vi "Graph Events.vi"() -> ()   [LabVIEW 2023]
doc: "This example shows some of the Waveform Graph events including cursor movement and changes in graph scale and plot properties."
panel:
  out "Iteration":i32
  out "Event Captured":string
  in  "Stop":bool
  out "Graph":dbl[](graph)
  # "Overview: Demonstrates several Events specific to graph indicators.\nInstructions:\n1. Run the VI and observe the Event Captured value when performing the following steps.\n2. Move the cursor within the graph.\n3. Click the image in the plot legend and select Common Plots, then select a new plot style.\n4. Change the minimum and/or maximum values in the X and Y scales.\n5. Click Stop to stop the VI."
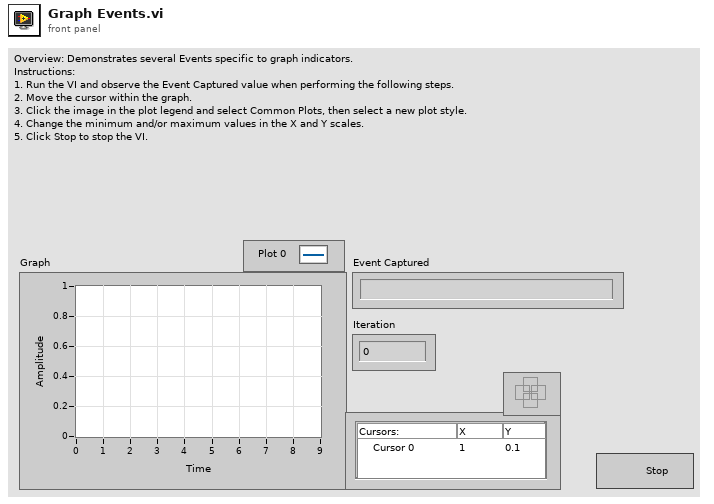
[diagram p1: front panel]
types:
  T1 = typedef "lveventtype.ctl" = enum32{"Null", "Timeout", "Annotation Menu Selection", "Annotation Menu Selection?", "App Instance Close", "App Instance Close?", "Autoscale Range Change", "Bookmark Info Change", "Cell Edit", "Cell Edit?", "Cursor Grab", "Cursor Grab?", "Cursor Menu Selection", "Cursor Menu Selection?", "Cursor Move", "Cursor Release", "Data Change", "Direction Change", "Display State Change", "Drag Ended", "Drag Enter", "Drag Leave", "Drag Over", "Drag Source Update", "Drag Starting", "Drag Starting?", "Drop", "Exec State Change", "Key Down", "Key Down?", "Key Repeat", "Key Repeat?", "Key Up", "Listbox Double Click", "Menu Activation?", "Menu Selection (App)", "Menu Selection? (App)", "Menu Selection (User)", "Mouse Down", "Mouse Down?", "Mouse Enter", "Mouse Leave", "Mouse Move", "Mouse Up", "Mouse Wheel", "NI Security User Change (App)", "Pane Size", "Panel Close", "Panel Close?", "Panel Resize", "Plot Attribute Change", "Scale Range Change", "Shortcut Menu Activation?", "Shortcut Menu Selection (App)", "Shortcut Menu Selection? (App)", "Shortcut Menu Selection (User)", "Tree Double Click", "Tree Drag", "Tree Drag?", "Tree Drop", "Tree Drop?", "Tree Item Close", "Tree Item Close?", "Tree Item Open", "Tree Item Open?", "User Event", "Value Change"}
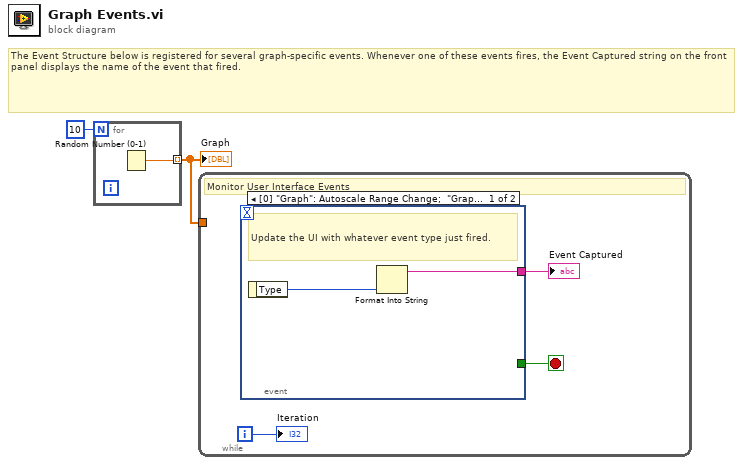
[diagram p0: block diagram]
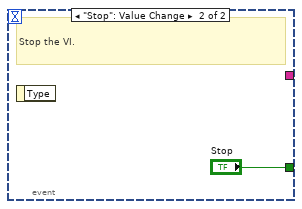
[diagram p2: hidden frame]
diagram:
  # "The Event Structure below is registered for several graph-specific events. Whenever one of these events fires, the Event Captured string on the front panel displays the name of the event that fired."
  n1 = for {
    N: 10 -> [_]
    tunnel: [w3] -> w1 mode=indexing
    n2 = Random Number (0-1)() -> (number: 0 to 1=w3:dbl)
  }
  "Graph" <- w1
  n3 = while {
    tunnel: w1 -> [_]
    i -> [w5]
    stop <- w6 stop-if-true
    # "Monitor User Interface Events"
    n4 = event shown="[0] \"Graph\": Autoscale Range Change;  \"Graph\": Plot Attribute Change;  \"Graph\": Scale Range Change;  \"Graph\": Cursor Grab;  \"Graph\": Cursor Move;  \"Graph\": Cursor Release" {
      selector: _ -> [_ _]
      dyn-events: _ -> [_ _]
      timeout: _ -> [_ _]
      tunnel: [_ "Stop"] -> w6
      tunnel: [w7 _] -> w4
      event "Graph": Autoscale Range Change; "Graph": Plot Attribute Change; "Graph": Scale Range Change; "Graph": Cursor Grab; "Graph": Cursor Move; "Graph": Cursor Release {
        # "Update the UI with whatever event type just fired."
        n5 = event-data() -> ("Type"=w8:T1)  [unwired: 1 in]
        n6 = Format Into String(w8) -> (resulting string=w7:string)  [unwired: 3 in, 1 out]
      }
      event "Stop": Value Change {
        # "Stop the VI."
        n7 = event-data() -> ()  [unwired: 1 in, 1 out]
      }
    }
    "Event Captured" <- w4
    "Iteration" <- w5
  }
